vi "RTTrapTest-09-12-2016.vi"() -> ()   [LabVIEW 2010]
uses:
  <vilib>/userDefined/High Color/nirio_resource_hc.ctl
  <vilib>/rvi/interface/nirviOpenFPGA/nirviOpenFPGA.xnode
  C:/Users/HAGAR-IV/Desktop/Zeugs/Johnny/pertrasgc fpga/FPGA-TrapTest-19-08-2016.vi
  <vilib>/rvi/ClientSDK/nirviWhatTheDeviceIsDoing.ctl
  <vilib>/rvi/interface/nirviReadWriteControl/nirviReadWriteControl.xnode
  <vilib>/rvi/interface/common/niFpgaNodeNameForErrorReporting.ctl
  <vilib>/rvi/errors/niLvFpgaWhatHappensToTopLevelVI.ctl
  <vilib>/rvi/interface/nirviMethod/nirviMethod.xnode
  <vilib>/rvi/interface/nirviCloseFPGA/nirviCloseFPGA.xnode
  <vilib>/FPGAPlugInAG/cRIO-9114/niLvFpga_Open_cRIO-9114.vi
  <vilib>/rvi/interface/common/dynamic/niFpgaDynamicAddResources.vi
  <vilib>/Utility/error.llb/Error Cluster From Error Code.vi
  <vilib>/rvi/errors/niLvFpgaAdjustHostInterfaceError.vi
  <vilib>/FPGAPlugInAG/Dynamic/niLvFpga_Close_Dynamic.vi
  NiFpgaLv.dll
panel:
  in  "Vorlaufzeit":dbl
  in  "Heizung aus":bool
  out "Uhr":dbl
  in  "Heizen&Starten":bool
  in  "Rampenende":dbl
  in  "T2":dbl
  in  "T1":dbl
  out "ThermoTemp":dbl
  out "PTTempTrap":dbl[](graph)
  in  "ThermoKoeff0":dbl=12.98
  in  "ThermoKoeff2":dbl=-136.78
  in  "ThermoKoeff1":dbl=1284.53
  in  "PTStirlingKoeff0":dbl=-248.3
  in  "PTStirlingKoeff2":dbl=2.42
  in  "PTStirlingKoeff1":dbl=108.05
  in  "SollwertTemp":dbl=50.0
  in  "R(T)Koeff0":dbl=7.31
  in  "R(T)Koeff2":dbl=5.2e-05
  in  "R(T)Koeff1":dbl=0.032
  out "TempTrap":dbl[](graph)
  in  "Löschen":bool
  out "SollwertSchpannung":dbl
  out "SollwertWidrschtond":dbl=8.43
  out "TempTrap":dbl
  in  "T(R)Koeff0":dbl=-236.6
  in  "T(R)Koeff2":dbl=-0.6
  in  "T(R)Koeff1":dbl=37.1
  out "WiderstandHeizdraht":dbl
  out "PTStirling":dbl format="%.2f"
  in  "Stirling":bool
  out "Thermo [V]":fxp<+/-,26,5> format="%.23g"
  in  "Messwerte":i32=10
  in  "Heizen":bool
  in  "5Van(us)":u16=5500
  in  "Periode(us)":u32=100000
  out "Messwert":fxp<+/-,27,6> format="%.23g"
  in  "Warten(us)":u16=5000
  in  "zwischenMesswerten(us)":u16=10
  in  "PID gains":T1={"proportional gain (Kc)"=5.0, "integral gain (Kc*Ts/Ti)"=0.0, "derivative gain (Kc*Td/Ts)"=0.0} {"proportional gain (Kc)" format="%.11g"; "integral gain (Kc*Ts/Ti)" format="%.11g"; "derivative gain (Kc*Td/Ts)" format="%.11g"}
  in  "stop":bool
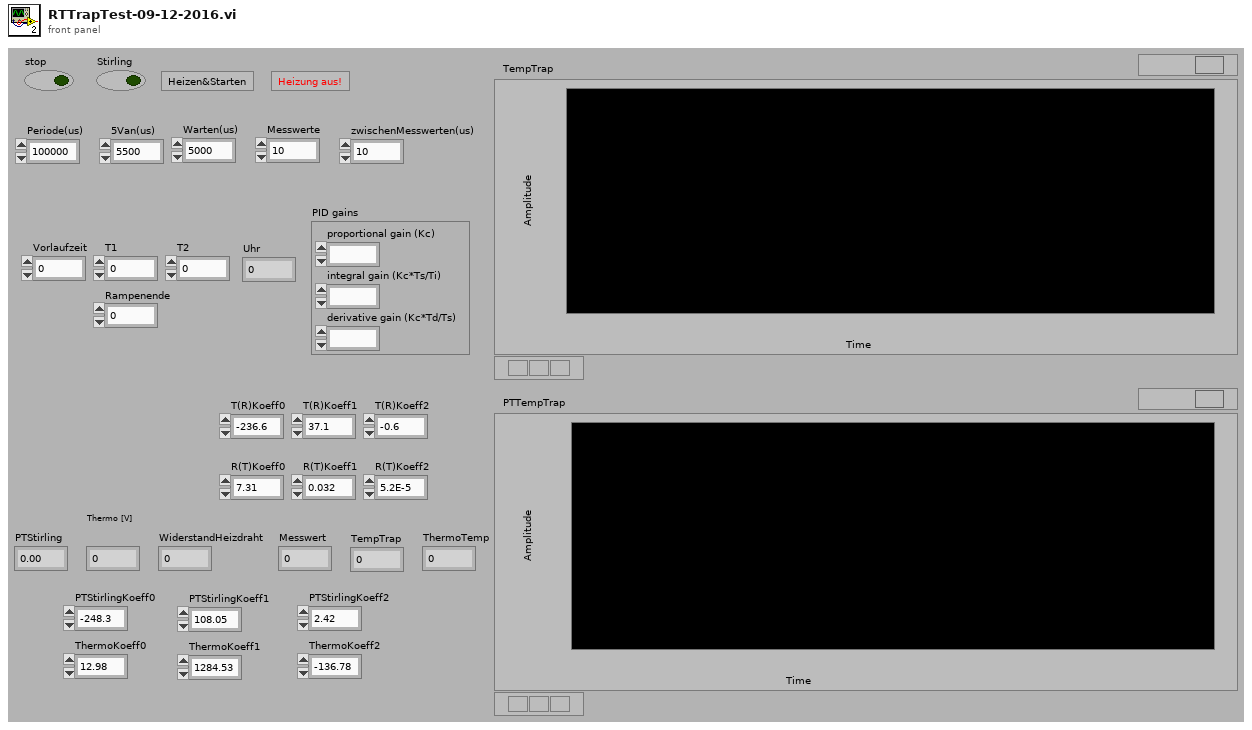
[diagram p1: front panel]
types:
  T1 = cluster{"proportional gain (Kc)":fxp<+/-,16,8>, "integral gain (Kc*Ts/Ti)":fxp<+/-,16,8>, "derivative gain (Kc*Td/Ts)":fxp<+/-,16,8>}
  T2 = typedef "niFpgaNodeNameForErrorReporting.ctl" = enum16{"Open FPGA VI Reference", "Read/Write Control", "Invoke Method: Abort", "Invoke Method: Acknowledge IRQ", "Invoke Method: Download", "Invoke Method: FIFO.Configure", "Invoke Method: FIFO.Read", "Invoke Method: FIFO.Start", "Invoke Method: FIFO.Stop", "Invoke Method: FIFO.Write", "Invoke Method: Reset", "Invoke Method: Run", "Invoke Method: Wait on IRQ", "Close FPGA VI Reference"}
  T3 = typedef "niLvFpgaWhatHappensToTopLevelVI.ctl" = enum16{"top level VI scripted behind XNode", "top level VI inlined behind XNode"}
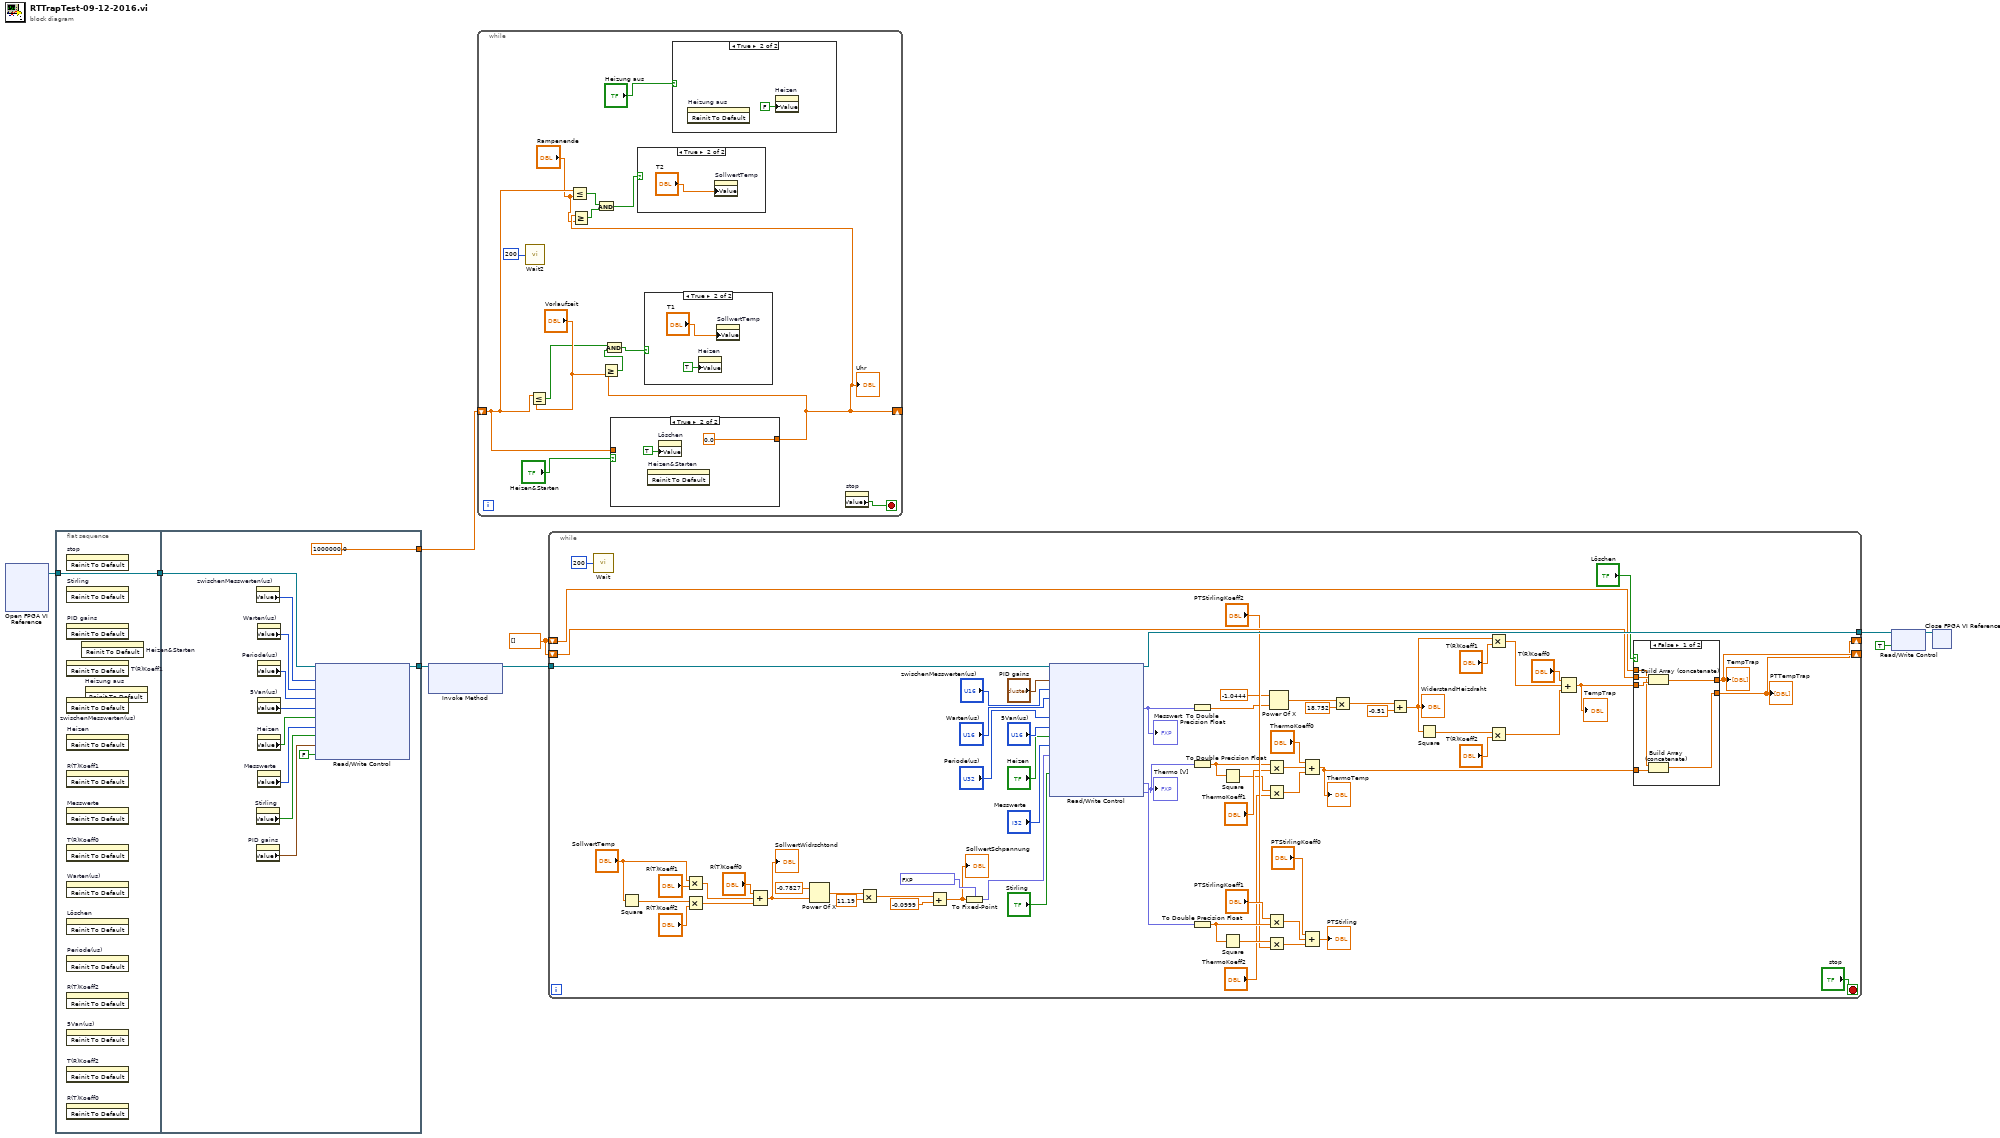
[diagram p0: block diagram]
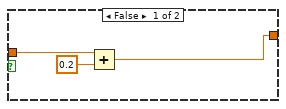
[diagram p5: hidden frame]
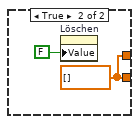
[diagram p6: hidden frame]
diagram:
  w2 = dbl[] []
  n1 = xnode "Open FPGA VI Reference"() -> ("FPGA VI Reference Out"=w9:refnum<k20>)  [unwired: 2 in, 1 out]
  n2 = flat-sequence {
    tunnel: w9 -> [w10]
    tunnel: [w10] -> w3
    tunnel: [w21] -> w8
    tunnel: w3 -> [w22]
    tunnel: [1000000.0] -> w1
    frame #0 {
      n3 = invoke on="stop" class="Bool (strict)" method="Reinit To Default"() -> ()  [unwired: 3 in, 3 out]
      n4 = invoke on="Stirling" class="Bool (strict)" method="Reinit To Default"() -> ()  [unwired: 3 in, 3 out]
      n5 = invoke on="PID gains" class="Clust (strict)" method="Reinit To Default"() -> ()  [unwired: 3 in, 3 out]
      n6 = invoke on="T(R)Koeff1" class="DigNum (strict)" method="Reinit To Default"() -> ()  [unwired: 3 in, 3 out]
      n7 = invoke on="zwischenMesswerten(us)" class="DigNum (strict)" method="Reinit To Default"() -> ()  [unwired: 3 in, 3 out]
      n8 = invoke on="Heizen" class="Bool (strict)" method="Reinit To Default"() -> ()  [unwired: 3 in, 3 out]
      n9 = invoke on="R(T)Koeff1" class="DigNum (strict)" method="Reinit To Default"() -> ()  [unwired: 3 in, 3 out]
      n10 = invoke on="Messwerte" class="DigNum (strict)" method="Reinit To Default"() -> ()  [unwired: 3 in, 3 out]
      n11 = invoke on="T(R)Koeff0" class="DigNum (strict)" method="Reinit To Default"() -> ()  [unwired: 3 in, 3 out]
      n12 = invoke on="Warten(us)" class="DigNum (strict)" method="Reinit To Default"() -> ()  [unwired: 3 in, 3 out]
      n13 = invoke on="Löschen" class="Bool (strict)" method="Reinit To Default"() -> ()  [unwired: 3 in, 3 out]
      n14 = invoke on="Periode(us)" class="DigNum (strict)" method="Reinit To Default"() -> ()  [unwired: 3 in, 3 out]
      n15 = invoke on="R(T)Koeff2" class="DigNum (strict)" method="Reinit To Default"() -> ()  [unwired: 3 in, 3 out]
      n16 = invoke on="5Van(us)" class="DigNum (strict)" method="Reinit To Default"() -> ()  [unwired: 3 in, 3 out]
      n17 = invoke on="T(R)Koeff2" class="DigNum (strict)" method="Reinit To Default"() -> ()  [unwired: 3 in, 3 out]
      n18 = invoke on="R(T)Koeff0" class="DigNum (strict)" method="Reinit To Default"() -> ()  [unwired: 3 in, 3 out]
      n19 = invoke on="Heizen&Starten" class="Bool" method="Reinit To Default"() -> ()  [unwired: 3 in, 3 out]
      n20 = invoke on="Heizung aus" class="Bool" method="Reinit To Default"() -> ()  [unwired: 3 in, 3 out]
    }
    frame #1 {
      n21 = property on="zwischenMesswerten(us)" class="DigNum (strict)"() -> ("Value"=w20:u16)  [unwired: 2 in, 2 out]
      n22 = property on="Stirling" class="Bool (strict)"() -> ("Value"=w14:bool)  [unwired: 2 in, 2 out]
      n23 = property on="PID gains" class="Clust (strict)"() -> ("Value"=w13:T1)  [unwired: 2 in, 2 out]
      n24 = property on="Warten(us)" class="DigNum (strict)"() -> ("Value"=w19:u16)  [unwired: 2 in, 2 out]
      n25 = property on="Periode(us)" class="DigNum (strict)"() -> ("Value"=w18:u32)  [unwired: 2 in, 2 out]
      n26 = property on="5Van(us)" class="DigNum (strict)"() -> ("Value"=w17:u16)  [unwired: 2 in, 2 out]
      n27 = property on="Heizen" class="Bool (strict)"() -> ("Value"=w16:bool)  [unwired: 2 in, 2 out]
      n28 = property on="Messwerte" class="DigNum (strict)"() -> ("Value"=w15:i32)  [unwired: 2 in, 2 out]
      n29 = xnode "Read/Write Control"("FPGA VI Reference In"=w22, "zwischenMesswerten(us)"=w20, "Warten(us)"=w19, "Periode(us)"=w18, "5Van(us)"=w17, "Heizen"=w16, "Messwerte"=w15, "Stirling"=w14, "PID gains"=w13, "stop"=FALSE) -> ("FPGA VI Reference Out"=w21:refnum<k20>)  [unwired: 1 in, 1 out]
    }
  }
  n30 = xnode "Invoke Method"("FPGA VI Reference In"=w8) -> ("FPGA VI Reference Out"=w7:refnum<k20>)  [unwired: 2 in, 1 out]
  n31 = while {
    shift-right: [w243] -> _
    shift-left: w1 -> [w244]
    stop <- w250 stop-if-true
    n32 = call "Wait2"("Count(mSec)"=u32 200) -> ()  [unwired: 1 out]
    n33 = Less Or Equal?(x=w244, y="Vorlaufzeit") -> (x <= y?=w246:bool)
    n34 = Less Or Equal?(x=w244, y="Rampenende") -> (x <= y?=w241:bool)
    n35 = case shown="True" "Heizen&Starten" {
      tunnel: w244 -> [w258 _]
      tunnel: [w256 0.0 ("t")] -> w243
      frame False {
        n36 = Add(x=w258, y=0.2) -> (x+y=w256:dbl)
      }
      frame True {
        n37 = invoke on="Heizen&Starten" class="Bool" method="Reinit To Default"() -> ()  [unwired: 3 in, 3 out]
        n38 = property on="Löschen" class="Bool (strict)"("Value"=TRUE ("Löschen")) -> ()  [unwired: 2 in, 2 out]
      }
    }
    "Uhr" <- w243
    n39 = Greater Or Equal?(x=w243, y="Rampenende") -> (x >= y?=w240:bool)
    n40 = And(x=w241, y=w240) -> (x .and. y?=w239:bool)
    n41 = Greater Or Equal?(x=w243, y="Vorlaufzeit") -> (x >= y?=w247:bool)
    n42 = And(x=w246, y=w247) -> (x .and. y?=w245:bool)
    n43 = case shown="True" w239 {
      frame False {
      }
      frame True {
        n44 = property on="SollwertTemp" class="DigNum (strict)"("Value"="T2") -> ()  [unwired: 2 in, 2 out]
      }
    }
    n45 = case shown="True" w245 {
      frame False {
      }
      frame True {
        n46 = property on="Heizen" class="Bool (strict)"("Value"=TRUE ("Heizen")) -> ()  [unwired: 2 in, 2 out]
        n47 = property on="SollwertTemp" class="DigNum (strict)"("Value"="T1") -> ()  [unwired: 2 in, 2 out]
      }
    }
    n48 = case shown="True" "Heizung aus" {
      frame False {
      }
      frame True {
        n49 = invoke on="Heizung aus" class="Bool" method="Reinit To Default"() -> ()  [unwired: 3 in, 3 out]
        n50 = property on="Heizen" class="Bool (strict)"("Value"=FALSE ("Heizen")) -> ()  [unwired: 2 in, 2 out]
      }
    }
    n51 = property on="stop" class="Bool (strict)"() -> ("Value"=w250:bool)  [unwired: 2 in, 2 out]
  }
  n52 = while {
    tunnel: w7 -> [w326]
    tunnel: [w324] -> w6
    shift-right: [w302] -> _
    shift-left: w2 -> [w304]
    shift-right: [w276] -> _
    shift-left: w2 -> [w285]
    stop <- "stop" stop-if-true
    n53 = call "Wait"("Count(mSec)"=u32 200) -> ()  [unwired: 1 out]
    n54 = Square(x="SollwertTemp") -> (x^2=w301:dbl)
    n55 = Multiply(x="SollwertTemp", y="R(T)Koeff1") -> (x*y=w296:dbl)
    n56 = Multiply(x=w301, y="R(T)Koeff2") -> (x*y=w295:dbl)
    n57 = Compound Arithmetic op=ADD("R(T)Koeff0", w296, w295) -> (w270:dbl)
    "SollwertWidrschtond" <- w270
    n58 = Power Of X(1:w270, 2:-0.7827 ("y")) -> (0:w266:dbl)
    n59 = Multiply(x=w266, y=11.19) -> (x*y=w264:dbl)
    n60 = Add(x=w264, y=-0.0999) -> (x+y=w262:dbl)
    "SollwertSchpannung" <- w262
    n61 = To Fixed-Point(fixed-point type=fxp<+/-,16,6> 0.0 ("setpoint"), number=w262) -> (fixed-point=w307:fxp<+/-,16,6>)
    n62 = xnode "Read/Write Control"("FPGA VI Reference In"=w326, "PID gains"="PID gains", "zwischenMesswerten(us)"="zwischenMesswerten(us)", "Warten(us)"="Warten(us)", "Periode(us)"="Periode(us)", "5Van(us)"="5Van(us)", "Heizen"="Heizen", "Messwerte"="Messwerte", "setpoint"=w307, "Stirling"="Stirling") -> ("FPGA VI Reference Out"=w324:refnum<k20>, "Messwert"=w309:fxp<+/-,27,6>, "PTStirling"=w287:fxp<+/-,26,5>, "Thermoelement"=w261:fxp<+/-,26,5>)  [unwired: 1 in, 2 out]
    "Messwert" <- w309
    "Thermo [V]" <- w261
    n63 = To Double Precision Float(number=w309) -> (double precision float=w269:dbl)
    n64 = To Double Precision Float(number=w261) -> (double precision float=w281:dbl)
    n65 = To Double Precision Float(number=w287) -> (double precision float=w293:dbl)
    n66 = Square(x=w281) -> (x^2=w280:dbl)
    n67 = Square(x=w293) -> (x^2=w292:dbl)
    n68 = Multiply(x=w281, y="ThermoKoeff1") -> (x*y=w282:dbl)
    n69 = Multiply(x=w280, y="ThermoKoeff2") -> (x*y=w278:dbl)
    n70 = Multiply(x="PTStirlingKoeff1", y=w293) -> (x*y=w289:dbl)
    n71 = Multiply(x=w292, y="PTStirlingKoeff2") -> (x*y=w288:dbl)
    n72 = Power Of X(1:w269, 2:-1.0444 ("x")) -> (0:w275:dbl)
    n73 = Compound Arithmetic op=ADD("ThermoKoeff0", w282, w278) -> (w277:dbl)
    "ThermoTemp" <- w277
    n74 = Compound Arithmetic op=ADD("PTStirlingKoeff0", w289, w288) -> (→"PTStirling":dbl)
    n75 = Multiply(x=w275, y=18.752) -> (x*y=w273:dbl)
    n76 = Add(x=w273, y=-0.51) -> (x+y=w271:dbl)
    "WiderstandHeizdraht" <- w271
    n77 = Square(x=w271) -> (x^2=w314:dbl)
    n78 = Multiply(x=w271, y="T(R)Koeff1") -> (x*y=w311:dbl)
    n79 = Multiply(x=w314, y="T(R)Koeff2") -> (x*y=w312:dbl)
    n80 = Compound Arithmetic op=ADD("T(R)Koeff0", w311, w312) -> (w305:dbl)
    "TempTrap" <- w305
    n81 = case shown="False" "Löschen" {
      tunnel: w305 -> [w332 _]
      tunnel: [w331 w333] -> w302
      tunnel: w304 -> [w330 _]
      tunnel: [w329 w333] -> w276
      tunnel: w285 -> [w328 _]
      tunnel: w277 -> [w327 _]
      frame False {
        n82 = Build Array (concatenate)(w330, w332) -> (w331:dbl[])
        n83 = Build Array (concatenate)(w328, w327) -> (w329:dbl[])
      }
      frame True {
        w333 = dbl[] []
        n84 = property on="Löschen" class="Bool (strict)"("Value"=FALSE ("Löschen")) -> ()  [unwired: 2 in, 2 out]
      }
    }
    "TempTrap" <- w302
    "PTTempTrap" <- w276
  }
  n85 = xnode "Read/Write Control"("FPGA VI Reference In"=w6, "stop"=TRUE) -> ("FPGA VI Reference Out"=w4:refnum<k20>)  [unwired: 1 in, 1 out]
  n86 = xnode "Close FPGA VI Reference"("FPGA VI Reference In"=w4) -> ()  [unwired: 1 in, 1 out]
